vi "Write Result.vi"(0 "Vector Charact Result Accessor in":refnum<class "Vector Charact Result Accessor.lvclass">, 5 "Charact Result":variant, 11 "error in":errorcluster) -> (4 "Vector Charact Result Accessor out":refnum<class "Vector Charact Result Accessor.lvclass">, 15 "error out":errorcluster)   [LabVIEW 2023, in "RFFixtureCharact.RFPM.lvlib" / "Vector Charact Result Accessor.lvclass"]
uses:
  Vector Charact Result Accessor.lvclass
  C:/rfcal/AuxTools/STSRFFixtureCharactUtility/Source/Code Modules/Fixture/RFPM/Charact Result Accessor/Base/Charact Result Accessor.lvclass
  Dependencies/HFNetworkAnalysis/Controls/SnPDataType.ctl
  Public/Base Classes/Vector/Vector Abstract Path/Type Definitions/Vector Charact Result.ctl
  Vector Charact Result Accessor.lvclass/Vector Charact Result Accessor.ctl
  Dependencies/HFNetworkAnalysis/NI_HFNetworkAnalysis.lvlib
  Public/Base Classes/Vector/Vector Abstract Path/Vector Abstract Path.lvclass
  Base/Charact Result Accessor.lvclass
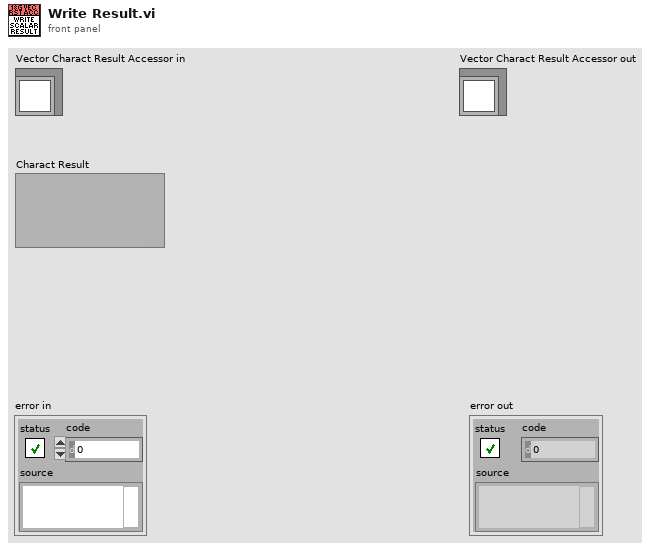
[diagram p1: front panel]
types:
  T1 = typedef "RFFixtureCharact.Public.lvlib/Vector Abstract Path.lvclass/Vector Charact Result.ctl" = cluster{"Port Power":dbl, "Frequency":dbl, "S Parameters":cdb[], "Out Of Limit":bool}
  T2 = typedef "NI_HFNetworkAnalysis.lvlib/SnPDataType.ctl" = enum16{"DB", "MA", "RI"}
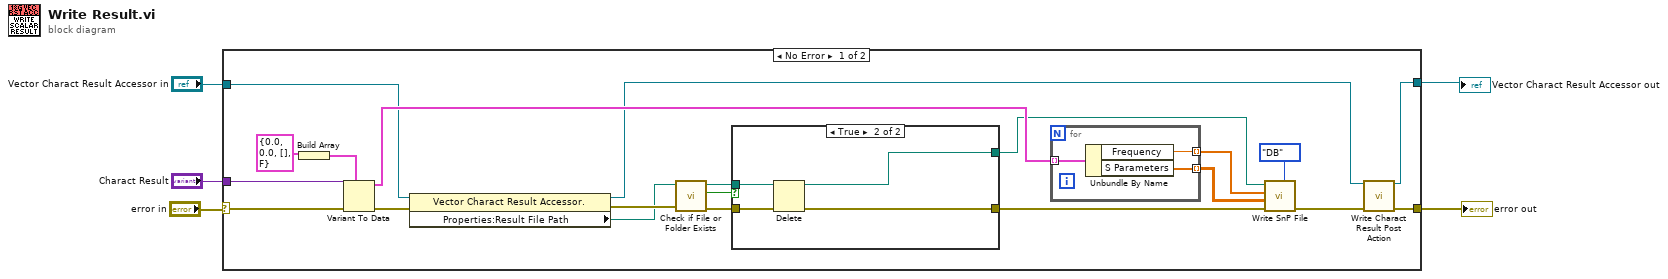
[diagram p0: block diagram]
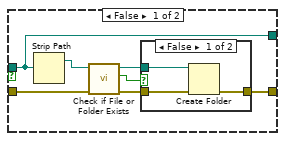
[diagram p2: hidden frame]
diagram:
  n1 = case shown="No Error" "error in" {
    selector: "error in" -> [w21 w46]
    tunnel: "Vector Charact Result Accessor in" -> [w16 w45]
    tunnel: [w13 w46] -> w2
    tunnel: "Charact Result" -> [w20 _]
    tunnel: [w11 w45] -> w1
    frame No Error {
      n2 = Build Array(T1 {"Port Power"=0.0, "Frequency"=0.0, "S Parameters"=[], "Out Of Limit"=FALSE} ("Cal Result")) -> (w22:T1[])
      n3 = Variant To Data(error in=w21, type=w22, Variant=w20) -> (data=w19:T1[], error out=w18:errorcluster)
      n4 = property class="Vector Charact Result Accessor."(reference=w16, error in=w18) -> (reference out=w12:refnum<class "Vector Charact Result Accessor.lvclass">, error out=w17:errorcluster, "Properties:Result File Path"=w15:path)
      n5 = call <vilib>:"Check if File or Folder Exists.vi"("error in (no error)"=w17, "path"=w15) -> ("error out"=w10:errorcluster, "file or folder exists?"=w9:bool, "dup path"=w8:path)  [unwired: 7 in]
      n6 = case shown="True" w9 {
        tunnel: [w28 w41] -> w7
        tunnel: [w27 w40] -> w6
        tunnel: w10 -> [w30 w39]
        tunnel: w8 -> [w27 w38]
        frame False {
          n7 = Strip Path(path=w27) -> (stripped path=w29:path)  [unwired: 1 out]
          n8 = call <vilib>:"Check if File or Folder Exists.vi"("error in (no error)"=w30, "path"=w29) -> ("error out"=w31:errorcluster, "file or folder exists?"=w33:bool, "dup path"=w32:path)  [unwired: 7 in]
          n9 = case shown="False" w33 {
            tunnel: w31 -> [w36 w37]
            tunnel: [w35 w37] -> w28
            tunnel: w32 -> [w34 _]
            frame False {
              n10 = Create Folder(path (use dialog)=w34, error in=w36) -> (error out=w35:errorcluster)  [unwired: 1 in, 2 out]
            }
            frame True {
            }
          }
        }
        frame True {
          n11 = Delete(path (use dialog)=w38, error in=w39) -> (deleted path=w40:path, error out=w41:errorcluster)  [unwired: 3 in, 1 out]
        }
      }
      n12 = for {
        tunnel: w19 -> [w44] mode=indexing
        tunnel: [w43] -> w26 mode=indexing
        tunnel: [w42] -> w25 mode=indexing
        n13 = Unbundle By Name(w44) -> ("Frequency"=w43:dbl, "S Parameters"=w42:cdb[])
      }
      n14 = call "Write SnP File.vi"("OutputDataType"=SnPDataType."DB", "error in (no error)"=w7, "S-parameters"=w25, "Frequencies (Hz)"=w26, "SnP File Path"=w6) -> ("error out"=w14:errorcluster)  [unwired: 6 in]
      n15 = call "Write Charact Result Post Action.vi"("Charact Result Accessor in"=w12, "error in"=w14) -> ("Charact Result Accessor out"=w11:refnum<class "Vector Charact Result Accessor.lvclass">, "error out"=w13:errorcluster)  [unwired: 12 in]
    }
    frame Error {
    }
  }
  "error out" <- w2
  "Vector Charact Result Accessor out" <- w1
